vi "nanocal -- nuclear schottky fit V8.vi"() -> ()   [LabVIEW 2021] (continued)
  T36 = typedef "eventvkey.ctl" = enum16{"ASCII", "Enter", "Return", "Shift", "Ctrl", "Alt", "Cmd", "Opt", "Caps", "NumLock", "Clear", "Break", "Up", "Down", "Left", "Right", "Insert", "Delete", "Home", "End", "PageUp", "PageDown", "Escape", "Help", "Pause", "ScrollLock", "F1", "F2", "F3", "F4", "F5", "F6", "F7", "F8", "F9", "F10", "F11", "F12", "F13", "F14", "F15", "F16", "F17", "F18", "F19", "F20", "F21", "F22", "F23", "F24", "Play", "VolumeUp", "VolumeDown", "Mute", "Two Byte Char"}
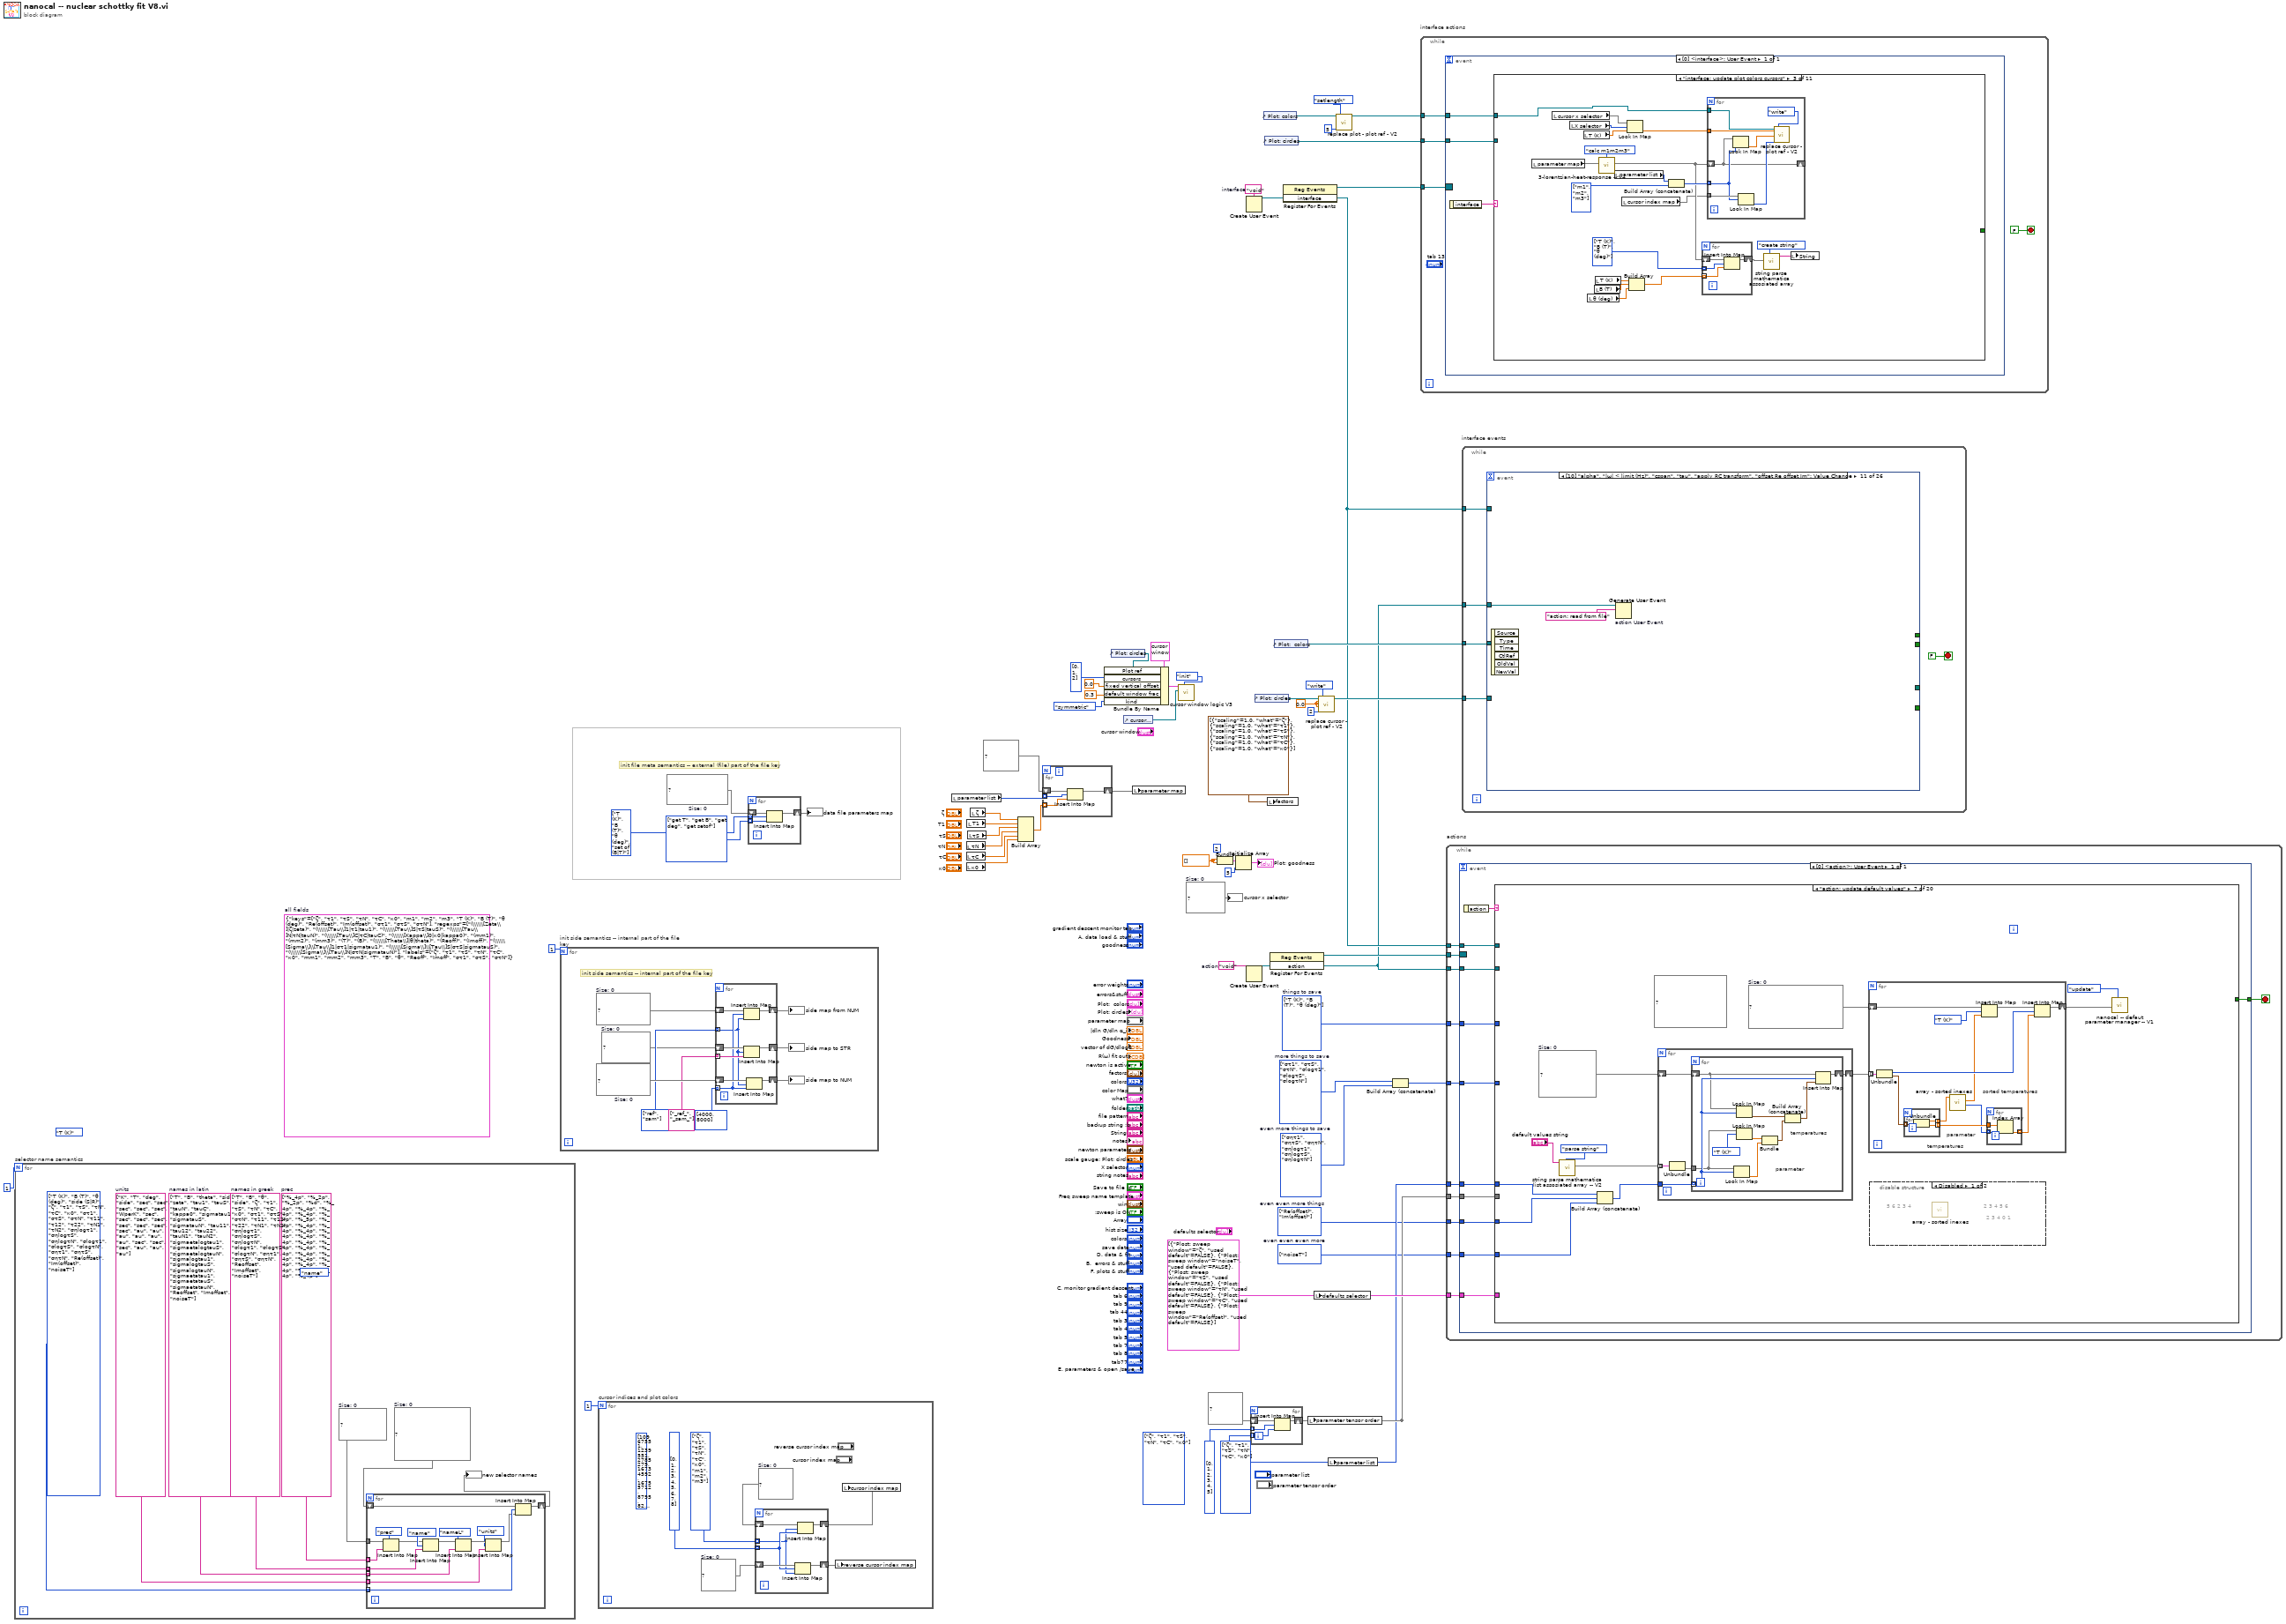
[diagram p0: block diagram]
diagram:
  w2 = T1[] [enum."noiseT"] items=["ζ", "τ1", "τS", "τN", "τC", "κ0", "m1", "m2", "m3", "T (K)", "B (T)", "θ (deg)", "side (S|R)", "set of (B|T)", "Re(offset)", "Im(offset)", "στ1", "στ1-", "στ1+", "στS", "στS-", "στS+", "στN", "στN-", "στN+", "τ11", "τ12", "τ21", "τ22", "τN1", "τN2", "σηlogτ1", "σηlogτS", "σηlogτN", "σlogτ1", "σlogτS", "σlogτN", "σητ1", "σητS", "σητN", "noiseT"]  # even even even more
  (unwired) 3-lorentzian-parameters."T (K)" ("Plost: sweep window")
  w3 = T1[] [enum."Re(offset)", enum."Im(offset)"] items=["ζ", "τ1", "τS", "τN", "τC", "κ0", "m1", "m2", "m3", "T (K)", "B (T)", "θ (deg)", "side (S|R)", "set of (B|T)", "Re(offset)", "Im(offset)", "στ1", "στ1-", "στ1+", "στS", "στS-", "στS+", "στN", "στN-", "στN+", "τ11", "τ12", "τ21", "τ22", "τN1", "τN2", "σηlogτ1", "σηlogτS", "σηlogτN", "σlogτ1", "σlogτS", "σlogτN", "σητ1", "σητS", "σητN", "noiseT"]  # even even more things
  w9 = T1[] [enum."σητ1", enum."σητS", enum."σητN", enum."σηlogτ1", enum."σηlogτS", enum."σηlogτN"] items=["ζ", "τ1", "τS", "τN", "τC", "κ0", "m1", "m2", "m3", "T (K)", "B (T)", "θ (deg)", "side (S|R)", "set of (B|T)", "Re(offset)", "Im(offset)", "στ1", "στ1-", "στ1+", "στS", "στS-", "στS+", "στN", "στN-", "στN+", "τ11", "τ12", "τ21", "τ22", "τN1", "τN2", "σηlogτ1", "σηlogτS", "σηlogτN", "σlogτ1", "σlogτS", "σlogτN", "σητ1", "σητS", "σητN", "noiseT"]  # even more things to save
  w12 = T1[] [enum."ζ", enum."τ1", enum."τS", enum."τN", enum."τC", enum."κ0"] items=["ζ", "τ1", "τS", "τN", "τC", "κ0", "m1", "m2", "m3", "T (K)", "B (T)", "θ (deg)", "side (S|R)", "set of (B|T)", "Re(offset)", "Im(offset)", "στ1", "στ1-", "στ1+", "στS", "στS-", "στS+", "στN", "στN-", "στN+", "τ11", "τ12", "τ21", "τ22", "τN1", "τN2", "σηlogτ1", "σηlogτS", "σηlogτN", "σlogτ1", "σlogτS", "σlogτN", "σητ1", "σητS", "σητN", "noiseT"]
  w16 = T1[] [enum."T (K)", enum."B (T)", enum."θ (deg)"] items=["ζ", "τ1", "τS", "τN", "τC", "κ0", "m1", "m2", "m3", "T (K)", "B (T)", "θ (deg)", "side (S|R)", "set of (B|T)", "Re(offset)", "Im(offset)", "στ1", "στ1-", "στ1+", "στS", "στS-", "στS+", "στN", "στN-", "στN+", "τ11", "τ12", "τ21", "τ22", "τN1", "τN2", "σηlogτ1", "σηlogτS", "σηlogτN", "σlogτ1", "σlogτS", "σlogτN", "σητ1", "σητS", "σητN", "noiseT"]  # things to save
  w11 = T1[] [enum."στ1", enum."στS", enum."στN", enum."σlogτ1", enum."σlogτS", enum."σlogτN"] items=["ζ", "τ1", "τS", "τN", "τC", "κ0", "m1", "m2", "m3", "T (K)", "B (T)", "θ (deg)", "side (S|R)", "set of (B|T)", "Re(offset)", "Im(offset)", "στ1", "στ1-", "στ1+", "στS", "στS-", "στS+", "στN", "στN-", "στN+", "τ11", "τ12", "τ21", "τ22", "τN1", "τN2", "σηlogτ1", "σηlogτS", "σηlogτN", "σlogτ1", "σlogτS", "σlogτN", "σητ1", "σητS", "σητN", "noiseT"]  # more things to save
  (unwired) T16 {"keys"=[enum."ζ", enum."τ1", enum."τS", enum."τN", enum."τC", enum."κ0", enum."m1", enum."m2", enum."m3", enum."T (K)", enum."B (T)", enum."θ (deg)", enum."Re(offset)", enum."Im(offset)", enum."στ1", enum."στS", enum."στN"], "regexps"=["(\\\\\\[Zeta\\]|ζ|zeta)", "(\\\\\\[Tau\\]1|τ1|tau1)", "(\\\\\\[Tau\\]S|τS|tauS)", "(\\\\\\[Tau\\]N|τN|tauN)", "(\\\\\\[Tau\\]C|τC|tauC)", "(\\\\\\[Kappa\\]0|κ0|kappa0)", "(mm1)", "(mm2)", "(mm3)", "(T)", "(B)", "(\\\\\\[Theta\\]|θ|theta)", "(Reoff)", "(Imoff)", "(\\\\\\[Sigma\\]\\[Tau\\]1|στ1|sigmatau1)", "(\\\\\\[Sigma\\]\\[Tau\\]S|στS|sigmatauS)", "(\\\\\\[Sigma\\]\\[Tau\\]N|στN|sigmatauN)"], "labels"=["ζ", "τ1", "τS", "τN", "τC", "κ0", "mm1", "mm2", "mm3", "T", "B", "θ", "Reoff", "Imoff", "στ1", "στS", "στN"]}  # all fields
  (unwired) 2 ("dimension size")
  w33 = T5 [{"Plost: sweep window"=enum."ζ", "used default"=FALSE}, {"Plost: sweep window"=enum."noiseT", "used default"=FALSE}, {"Plost: sweep window"=enum."τS", "used default"=FALSE}, {"Plost: sweep window"=enum."τN", "used default"=FALSE}, {"Plost: sweep window"=enum."τC", "used default"=FALSE}, {"Plost: sweep window"=enum."Re(offset)", "used default"=FALSE}] ("parameter 2")
  w34 = T13[] [enum."get T", enum."get B", enum."get deg", enum."get setof"] items=["rewrite", "parse", "force pattern", "uniquenum", "get T", "get B", "get ind", "get deg", "get name", "get folder", "get extension", "get basename", "get side", "get setof", "getID", "getIDStock"]
  w36 = map{T1, T13} {}  # Size: 0
  w35 = T1[] [enum."T (K)", enum."B (T)", enum."θ (deg)", enum."set of (B|T)"] items=["ζ", "τ1", "τS", "τN", "τC", "κ0", "m1", "m2", "m3", "T (K)", "B (T)", "θ (deg)", "side (S|R)", "set of (B|T)", "Re(offset)", "Im(offset)", "στ1", "στ1-", "στ1+", "στS", "στS-", "στS+", "στN", "στN-", "στN+", "τ11", "τ12", "τ21", "τ22", "τN1", "τN2", "σηlogτ1", "σηlogτS", "σηlogτN", "σlogτ1", "σlogτS", "σlogτN", "σητ1", "σητS", "σητN", "noiseT"]
  w40 = dbl[] []
  (unwired) T1[] [enum."ζ", enum."τ1", enum."τS", enum."τN", enum."τC", enum."κ0"] items=["ζ", "τ1", "τS", "τN", "τC", "κ0", "m1", "m2", "m3", "T (K)", "B (T)", "θ (deg)", "side (S|R)", "set of (B|T)", "Re(offset)", "Im(offset)", "στ1", "στ1-", "στ1+", "στS", "στS-", "στS+", "στN", "στN-", "στN+", "τ11", "τ12", "τ21", "τ22", "τN1", "τN2", "σηlogτ1", "σηlogτS", "σηlogτN", "σlogτ1", "σlogτS", "σlogτN", "σητ1", "σητS", "σητN", "noiseT"]
  w43 = map{T1, dbl} {}  # Size: 0
  w44 = 0.0 ("new X")
  w57 = "void"  # interface
  w58 = "void"  # action
  # "init file meta semantics -- external (file) part of the file key"
  n1 = for "selector name semantics" {
    N: 1 -> [_]
    w60 = string[] ["%_4p", "%_2p", "%_2p", "%d", "%_4p", "%_4p", "%_4p", "%_4p", "%_4p", "%_5p", "%_4p", "%_4p", "%_4p", "%_4p", "%_4p", "%_4p", "%_4p", "%_4p", "%_4p", "%_4p", "%_4p", "%_4p", "%_4p", "%_4p", "%_4p", "%_4p", "%_4p", "%_4p", "%_4p", "%_4p"]  # prec
    w64 = map{T14, string} {}  # Size: 0
    (unwired) nameformattingitem."name" ("name formatting item")
    w62 = string[] ["K", "T", "deg", "side", "sec", "sec", "sec", "sec", "sec", "WperK", "sec", "sec", "sec", "sec", "sec", "sec", "sec", "sec", "au", "au", "au", "au", "au", "au", "sec", "sec", "sec", "au", "au", "au"]  # units
    w65 = string[] ["T", "B", "theta", "side", "zeta", "tau1", "tauS", "tauN", "tauC", "kappa0", "sigmatau1", "sigmatauS", "sigmatauN", "tau11", "tau12", "tau22", "tauN1", "tauN2", "sigmaetalogtau1", "sigmaetalogtauS", "sigmaetalogtauN", "sigmalogtau1", "sigmalogtauS", "sigmalogtauN", "sigmaetatau1", "sigmaetatauS", "sigmaetatauN", "Reoffset", "Imoffset", "noiseT"]  # names in latin
    w63 = string[] ["T", "B", "θ", "side", "ζ", "τ1", "τS", "τN", "τC", "κ0", "στ1", "στS", "στN", "τ11", "τ12", "τ22", "τN1", "τN2", "σηlogτ1", "σηlogτS", "σηlogτN", "σlogτ1", "σlogτS", "σlogτN", "σητ1", "σητS", "σητN", "Reoffset", "Imoffset", "noiseT"]  # names in greek
    w67 = map{T1, map{T14, string}} {}  # Size: 0
    w66 = T1[] [enum."T (K)", enum."B (T)", enum."θ (deg)", enum."side (S|R)", enum."ζ", enum."τ1", enum."τS", enum."τN", enum."τC", enum."κ0", enum."στ1", enum."στS", enum."στN", enum."τ11", enum."τ12", enum."τ22", enum."τN1", enum."τN2", enum."σηlogτ1", enum."σηlogτS", enum."σηlogτN", enum."σlogτ1", enum."σlogτS", enum."σlogτN", enum."σητ1", enum."σητS", enum."σητN", enum."Re(offset)", enum."Im(offset)", enum."noiseT"] items=["ζ", "τ1", "τS", "τN", "τC", "κ0", "m1", "m2", "m3", "T (K)", "B (T)", "θ (deg)", "side (S|R)", "set of (B|T)", "Re(offset)", "Im(offset)", "στ1", "στ1-", "στ1+", "στS", "στS-", "στS+", "στN", "στN-", "στN+", "τ11", "τ12", "τ21", "τ22", "τN1", "τN2", "σηlogτ1", "σηlogτS", "σηlogτN", "σlogτ1", "σlogτS", "σlogτN", "σητ1", "σητS", "σητN", "noiseT"]
    n2 = for {
      shift-right: [w82] -> w61
      shift-left: w67 -> [w83]
      tunnel: w65 -> [w73] mode=indexing
      tunnel: w66 -> [w81] mode=indexing
      tunnel: w64 -> [w71]
      tunnel: w63 -> [w72] mode=indexing
      tunnel: w62 -> [w74] mode=indexing
      tunnel: w60 -> [w70] mode=indexing
      n3 = Insert Into Map(map in=w71, key=nameformattingitem."prec", value=w70) -> (map out=w69:map{T14, string})  [unwired: 2 out]
      n4 = Insert Into Map(map in=w69, key=nameformattingitem."name", value=w72) -> (map out=w80:map{T14, string})  [unwired: 2 out]
      n5 = Insert Into Map(map in=w80, key=nameformattingitem."nameL" ("name formatting item"), value=w73) -> (map out=w79:map{T14, string})  [unwired: 2 out]
      n6 = Insert Into Map(map in=w79, key=nameformattingitem."units" ("name formatting item"), value=w74) -> (map out=w78:map{T14, string})  [unwired: 2 out]
      n7 = Insert Into Map(map in=w83, key=w81, value=w78) -> (map out=w82:map{T1, map{T14, string}})  [unwired: 2 out]
    }
    "new selector names" <- w61
  }
  n8 = for "init side semantics -- internal part of the file key" {
    N: 1 -> [_]
    w85 = map{i32, T9} {}  # Size: 0
    w87 = map{T9, string} {}  # Size: 0
    w88 = T9[] [enum."ref", enum."sam"] items=["sam", "ref"]
    w92 = map{T9, i32} {}  # Size: 0
    # "init side semantics -- internal part of the file key"
    n9 = for {
      shift-right: [w100] -> w89
      shift-left: w92 -> [w101]
      tunnel: string[] ["_ref_", "_sam_"] -> [w97] mode=indexing
      tunnel: i32[] [4000, 8000] -> [w94] mode=indexing
      tunnel: w88 -> [w93] mode=indexing
      shift-right: [w98] -> w86
      shift-left: w87 -> [w99]
      shift-right: [w95] -> w84
      shift-left: w85 -> [w96]
      n10 = Insert Into Map(map in=w96, key=w94, value=w93) -> (map out=w95:map{i32, T9})  [unwired: 2 out]
      n11 = Insert Into Map(map in=w99, key=w93, value=w97) -> (map out=w98:map{T9, string})  [unwired: 2 out]
      n12 = Insert Into Map(map in=w101, key=w93, value=w94) -> (map out=w100:map{T9, i32})  [unwired: 2 out]
    }
    "side map from NUM" <- w84
    "side map to STR" <- w86
    "side map to NUM" <- w89
  }
  n13 = for "cursor indices and plot colors" {
    N: 1 -> [_]
    w103 = map{i32, T1} {}  # Size: 0
    (unwired) u32[] [10967551, 1239551, 2785279, 16734592, 16755712, 8795, 8285330, 9272482, 9204890]
    w107 = map{T1, i32} {}  # Size: 0
    w104 = T1[] [enum."ζ", enum."τ1", enum."τS", enum."τN", enum."τC", enum."κ0", enum."m1", enum."m2", enum."m3"] items=["ζ", "τ1", "τS", "τN", "τC", "κ0", "m1", "m2", "m3", "T (K)", "B (T)", "θ (deg)", "side (S|R)", "set of (B|T)", "Re(offset)", "Im(offset)", "στ1", "στ1-", "στ1+", "στS", "στS-", "στS+", "στN", "στN-", "στN+", "τ11", "τ12", "τ21", "τ22", "τN1", "τN2", "σηlogτ1", "σηlogτS", "σηlogτN", "σlogτ1", "σlogτS", "σlogτN", "σητ1", "σητS", "σητN", "noiseT"]
    n14 = for {
      shift-right: [w112] -> w105
      shift-left: w107 -> [w113]
      tunnel: w104 -> [w108] mode=indexing
      tunnel: i32[] [0, 1, 2, 3, 4, 5, 6, 7, 8] -> [w109] mode=indexing
      shift-right: [w110] -> w102
      shift-left: w103 -> [w111]
      n15 = Insert Into Map(map in=w111, key=w109, value=w108) -> (map out=w110:map{i32, T1})  [unwired: 2 out]
      n16 = Insert Into Map(map in=w113, key=w108, value=w109) -> (map out=w112:map{T1, i32})  [unwired: 2 out]
    }
    n17 = local write "reverse cursor index map"(w102) -> ()
    n18 = local write "cursor index map"(w105) -> ()
  }
  n19 = for {
    shift-right: [w116] -> w37
    shift-left: w36 -> [w117]
    tunnel: w35 -> [w115] mode=indexing
    tunnel: w34 -> [w114] mode=indexing
    n20 = Insert Into Map(map in=w117, key=w115, value=w114) -> (map out=w116:map{T1, T13})  [unwired: 2 out]
  }
  "data file parameters map" <- w37
  n21 = local read "parameter list"() -> (w1:T1[])
  n22 = local read "τN"() -> (w25:dbl)
  n23 = local read "τC"() -> (w26:dbl)
  n24 = local read "κ0"() -> (w27:dbl)
  n25 = local read "T1"() -> (w23:dbl)
  n26 = local read "τS"() -> (w24:dbl)
  n27 = local read "ζ"() -> (w22:dbl)
  n28 = Build Array(w22, w23, w24, w25, w26, w27) -> (w28:dbl[])
  n29 = for {
    shift-right: [w120] -> w29
    shift-left: map{T1, dbl} {} ("Map IN") -> [w121]
    tunnel: w1 -> [w119] mode=indexing
    tunnel: w28 -> [w118] mode=indexing
    n30 = Insert Into Map(map in=w121, key=w119, value=w118) -> (map out=w120:map{T1, dbl})  [unwired: 2 out]
  }
  n31 = control-ref of="Plot: circles"() -> (w49:refnum<vi>)
  n32 = Bundle By Name(cluster=T12 {"left"=0.0, "right "=0.0, "center"=0.0, "window"=0.0, "cursors"=[], "relative"=0, "absolute"=0, "fixed vertical offset"=0.0, "vertical offset"=0.0, "skew"=0.0, "default window frac"=0.0, "kind"=enum."symmetric", "skew.left"=0.0, "skew.right"=0.0, "Plot ref"=refnum, "wing order"=enum."forw"} ("cursor bracket: All, data window"), "Plot ref"=w49, "cursors"=i32[] [0, 1, 2], "fixed vertical offset"=0.0, "default window frac"=0.3 ("fixed vertical offset"), "kind"=enum16{"symmetric", "skewed", "fancy"}."symmetric") -> (w52:T12)
  n33 = control-ref of="cursor window"() -> (w48:refnum<vi>)
  n34 = local write "parameter map"(w29) -> ()
  n35 = call "cursor window logic V3.vi"("cursor window action"=cursor_window_action."init", "cursor window in"=w48, "cursor window init"=w52) -> ()  [unwired: 7 in, 2 out]
  n36 = Bundle(w40, w40) -> (w17:cluster{dbl[], dbl[]})  [unwired: 1 in]
  n37 = Initialize Array(w17, 5 ("dimension size")) -> (→"Plot: goodness":cluster{dbl[], dbl[]}[])
  n38 = Create User Event(user event datatype=w57) -> (user event=w19:refnum<user-event>)  [unwired: 1 in, 1 out]
  n39 = Create User Event(user event datatype=w58) -> (user event=w18:refnum<user-event>)  [unwired: 1 in, 1 out]
  n40 = for {
    tunnel: w12 -> [w122] mode=indexing
    shift-right: [w124] -> w13
    shift-left: map{i32, T1} {} ("parameters IN") -> [w125]
    tunnel: i32[] [0, 1, 2, 3, 4, 5] -> [w123] mode=indexing
    n41 = Insert Into Map(map in=w125, key=w123, value=w122) -> (map out=w124:map{i32, T1})  [unwired: 2 out]
  }
  n42 = control-ref of="Plot: circles"() -> (w45:refnum<vi>)
  n43 = control-ref of="Plot: colors"() -> (w5:refnum<vi>)
  n44 = control-ref of="Plot: circles"() -> (w6:refnum<vi>)
  n45 = local write "factors"(cluster{"scaling":dbl, "what":T1}[] [{"scaling"=1.0, "what"=enum."ζ"}, {"scaling"=1.0, "what"=enum."τ1"}, {"scaling"=1.0, "what"=enum."τS"}, {"scaling"=1.0, "what"=enum."τN"}, {"scaling"=1.0, "what"=enum."τC"}, {"scaling"=1.0, "what"=enum."κ0"}]) -> ()
  n46 = register-events(w18) -> (reference out=w59:refnum<event-registration>)  [unwired: 2 in, 1 out]
  n47 = control-ref of="Plot:  colors"() -> (w42:refnum<vi>)
  n48 = register-events(w19) -> (reference out=w20:refnum<event-registration>)  [unwired: 2 in, 1 out]
  n49 = local write "parameter tensor order"(w13) -> ()
  n50 = local write "defaults selector"(w33) -> ()
  n51 = call "replace cursor - plot ref - V2.vi"("Plot ref in"=w45, "new X"=w44, "new  Y"=w44, "cursor index"=2, "cursor action"=cursor_action."write") -> ()  [unwired: 11 in, 4 out]
  n52 = local write "parameter list"(w12) -> ()
  n53 = call "replace plot - plot ref - V2.vi"("Plot ref in"=w5, "plot index"=5, "cursor action"=cursor_action."setlength") -> ("Plot ref out"=w4:refnum<vi>)  [unwired: 12 in, 4 out]
  n54 = Build Array (concatenate)(w11, w9) -> (w10:T1[])
  n55 = while "interface actions" {
    tunnel: w20 -> [w129]
    tunnel: w4 -> [w128]
    tunnel: w6 -> [w127]
    stop <- FALSE stop-if-true
    n56 = event shown="[0] <interface>: User Event" {
      selector: w129 -> [_]
      dyn-events: _ -> [_]
      timeout: _ -> [_]
      tunnel: w128 -> [w131]
      tunnel: w127 -> [w130]
      event User Event {
        n57 = event-data() -> ("interface"=w132:string)  [unwired: 1 in]
        n58 = case shown="\"interface: update plot colors cursors\"" w132 {
          tunnel: [_ _ _ _ _ _ _ _ _ _ TRUE] -> _
          tunnel: w131 -> [_ _ w153 w185 _ _ w236 w307 _ _ _]
          tunnel: w130 -> [_ _ _ _ w203 _ _ _ _ _ _]
          frame "void", Default {
          }
          frame "interface: reset colors" {
            w139 = map{T1, u32} {}  # Size: 0
            n59 = local read "parameter list"() -> (w142:T1[])
            n60 = local read "colors"() -> (w140:u32[])
            n61 = for {
              shift-right: [w151] -> w141
              shift-left: w139 -> [w152]
              tunnel: w142 -> [w150] mode=indexing
              tunnel: w140 -> [w149] mode=indexing
              n62 = Insert Into Map(map in=w152, key=w150, value=w149) -> (map out=w151:map{T1, u32})  [unwired: 2 out]
            }
            n63 = local write "color Map"(w141) -> ()
            n64 = Look In Map(map=w141, key=3-lorentzian-parameters."ζ" ("Plost: sweep window")) -> (value=w143:u32)  [unwired: 1 in, 1 out]
            n65 = Look In Map(map=w141, key=3-lorentzian-parameters."τ1" ("Plost: sweep window")) -> (value=w144:u32)  [unwired: 1 in, 1 out]
            n66 = Look In Map(map=w141, key=3-lorentzian-parameters."τS" ("Plost: sweep window")) -> (value=w145:u32)  [unwired: 1 in, 1 out]
            n67 = Look In Map(map=w141, key=3-lorentzian-parameters."τN" ("Plost: sweep window")) -> (value=w146:u32)  [unwired: 1 in, 1 out]
            n68 = Look In Map(map=w141, key=3-lorentzian-parameters."τC" ("Plost: sweep window")) -> (value=w147:u32)  [unwired: 1 in, 1 out]
            n69 = Look In Map(map=w141, key=3-lorentzian-parameters."κ0" ("Plost: sweep window")) -> (value=w148:u32)  [unwired: 1 in, 1 out]
            n70 = property on="ζ" class="Slide (strict)"("Fill Color"=w143) -> ()  [unwired: 2 in, 2 out]
            n71 = property on="T1" class="Slide (strict)"("Fill Color"=w144) -> ()  [unwired: 2 in, 2 out]
            n72 = property on="τS" class="Slide (strict)"("Fill Color"=w145) -> ()  [unwired: 2 in, 2 out]
            n73 = property on="τN" class="Slide (strict)"("Fill Color"=w146) -> ()  [unwired: 2 in, 2 out]
            n74 = property on="τC" class="Slide (strict)"("Fill Color"=w147) -> ()  [unwired: 2 in, 2 out]
            n75 = property on="κ0" class="Slide (strict)"("Fill Color"=w148) -> ()  [unwired: 2 in, 2 out]
          }
          frame "interface: update plot colors cursors" {
            w158 = T1[] [enum."m1", enum."m2", enum."m3"] items=["ζ", "τ1", "τS", "τN", "τC", "κ0", "m1", "m2", "m3", "T (K)", "B (T)", "θ (deg)", "side (S|R)", "set of (B|T)", "Re(offset)", "Im(offset)", "στ1", "στ1-", "στ1+", "στS", "στS-", "στS+", "στN", "στN-", "στN+", "τ11", "τ12", "τ21", "τ22", "τN1", "τN2", "σηlogτ1", "σηlogτS", "σηlogτN", "σlogτ1", "σlogτS", "σlogτN", "σητ1", "σητS", "σητN", "noiseT"]
            w156 = T1[] [enum."T (K)", enum."B (T)", enum."θ (deg)"] items=["ζ", "τ1", "τS", "τN", "τC", "κ0", "m1", "m2", "m3", "T (K)", "B (T)", "θ (deg)", "side (S|R)", "set of (B|T)", "Re(offset)", "Im(offset)", "στ1", "στ1-", "στ1+", "στS", "στS-", "στS+", "στN", "στN-", "στN+", "τ11", "τ12", "τ21", "τ22", "τN1", "τN2", "σηlogτ1", "σηlogτS", "σηlogτN", "σlogτ1", "σlogτS", "σlogτN", "σητ1", "σητS", "σητN", "noiseT"]
            n76 = local read "parameter map"() -> (w171:map{T1, dbl})
            n77 = local read "cursor x selector"() -> (w159:map{T1, dbl})
            n78 = local read "X selector"() -> (w160:T1)
            n79 = local read "T (K)"() -> (w161:dbl)
            n80 = local read "θ (deg)"() -> (w166:dbl)
            n81 = local read "B (T)"() -> (w165:dbl)
            n82 = local read "T (K)"() -> (w164:dbl)
            n83 = call "3-lorentzian-heat-response -- V4.vi"("action"=3-lorentzian-heat-response_action."calc m1m2m3", "Map IN"=w171) -> ("Map OUT"=w167:map{T1, dbl})  [unwired: 7 in, 2 out]
            n84 = local read "parameter list"() -> (w172:T1[])
            n85 = local read "cursor index map"() -> (w163:map{T1, i32})
            n86 = Look In Map(map=w159, key=w160, default value=w161) -> (value=w162:dbl)  [unwired: 1 out]
            n87 = Build Array(w164, w165, w166) -> (w154:dbl[])
            n88 = Build Array (concatenate)(w172, w158) -> (w170:T1[])
            n89 = for {
              shift-right: [w175] -> w168
              shift-left: w167 -> [w176]
              tunnel: w156 -> [w174] mode=indexing
              tunnel: w154 -> [w173] mode=indexing
              n90 = Insert Into Map(map in=w176, key=w174, value=w173) -> (map out=w175:map{T1, dbl})  [unwired: 2 out]
            }
            n91 = for {
              tunnel: w162 -> [w184]
              tunnel: w153 -> [w183]
              tunnel: w170 -> [w179] mode=indexing
              tunnel: w163 -> [w181]
              shift-right: [w178] -> _
              shift-left: w167 -> [w178]
              n92 = Look In Map(map=w178, key=w179) -> (value=w177:dbl)  [unwired: 1 in, 1 out]
              n93 = Look In Map(map=w181, key=w179) -> (value=w180:i32)  [unwired: 1 in, 1 out]
              n94 = call "replace cursor - plot ref - V2.vi"("Plot ref in"=w183, "new X"=w184, "new  Y"=w177, "cursor index"=w180, "cursor action"=cursor_action."write") -> ()  [unwired: 11 in, 4 out]
            }
            n95 = call "string parse mathematica assosiated array.vi"("action"=mathematica_string_map_action."create string" ("derivative"), "map IN"=w168) -> ("String OUT"=w169:string)  [unwired: 8 in, 1 out]
            n96 = local write "String"(w169) -> ()
          }
          frame "interface: plot colors update m1m2m3 cursors" {
            w186 = T1[] [enum."m1", enum."m2", enum."m3"] items=["ζ", "τ1", "τS", "τN", "τC", "κ0", "m1", "m2", "m3", "T (K)", "B (T)", "θ (deg)", "side (S|R)", "set of (B|T)", "Re(offset)", "Im(offset)", "στ1", "στ1-", "στ1+", "στS", "στS-", "στS+", "στN", "στN-", "στN+", "τ11", "τ12", "τ21", "τ22", "τN1", "τN2", "σηlogτ1", "σηlogτS", "σηlogτN", "σlogτ1", "σlogτS", "σlogτN", "σητ1", "σητS", "σητN", "noiseT"]
            n97 = local read "parameter map"() -> (w194:map{T1, dbl})
            n98 = call "3-lorentzian-heat-response -- V4.vi"("action"=3-lorentzian-heat-response_action."calc m1m2m3", "Map IN"=w194) -> ("Map OUT"=w193:map{T1, dbl})  [unwired: 7 in, 2 out]
            n99 = local read "cursor x selector"() -> (w188:map{T1, dbl})
            n100 = local read "X selector"() -> (w189:T1)
            n101 = local read "cursor index map"() -> (w192:map{T1, i32})
            n102 = local read "T (K)"() -> (w190:dbl)
            n103 = Look In Map(map=w188, key=w189, default value=w190) -> (value=w191:dbl)  [unwired: 1 out]
            n104 = for {
              tunnel: w191 -> [w202]
              tunnel: w186 -> [w198] mode=indexing
              tunnel: w192 -> [w200]
              shift-right: [w197] -> _
              shift-left: w193 -> [w197]
              tunnel: w185 -> [w195]
              n105 = Look In Map(map=w197, key=w198) -> (value=w196:dbl)  [unwired: 1 in, 1 out]
              n106 = Look In Map(map=w200, key=w198) -> (value=w199:i32)  [unwired: 1 in, 1 out]
              n107 = call "replace cursor - plot ref - V2.vi"("Plot ref in"=w195, "new X"=w202, "new  Y"=w196, "cursor index"=w199, "cursor action"=cursor_action."write") -> ()  [unwired: 11 in, 4 out]
            }
          }
          frame "interface: update circle fit plot" {
            n108 = for {
              N: 1 -> [_]
              tunnel: w203 -> [w206]
              n109 = local read "update  ind"() -> (w208:i32)
              n110 = local read "vector of dG/dlogα"() -> (w210:dbl[])
              n111 = Increment(x=w208) -> (x+1=w207:i32)
              n112 = local read "R(ω) fit out"() -> (w216:cdb[])
              n113 = Square(x=w210) -> (x^2=w205:dbl[])
              n114 = local write "update  ind"(w207) -> ()
              n115 = Complex To Re/Im(x + iy=w216) -> (x=w214:dbl[], y=w215:dbl[])
              n116 = Add Array Elements(numeric array=w205) -> (sum=w211:dbl)
              n117 = call "replace plot - plot ref - V2.vi"("Plot ref in"=w206, "Array X IN"=w214, "Array Y IN"=w215, "plot index"=enum16{"data R(ω)", "fit R(ω)"}."fit R(ω)" ("Plost: sweep window"), "cursor action"=cursor_action."write") -> ()  [unwired: 10 in, 5 out]
              n118 = Square Root(x=w211) -> (sqrt(x)=w209:dbl)
              n119 = local write "|dln G/dln α_i |"(w209) -> ()
            }
          }
          frame "interface: update curvature plot" {
            n120 = local read "newton parameters"() -> (w219:T2)
            n121 = local read "error weights"() -> (w218:T4)
            n122 = Bundle By Name(cluster=w219, "weighting"=w218) -> (w217:T2)
            n123 = case shown="True" "update errors as you fit" {
              tunnel: w217 -> [_ w225]
              frame False {
              }
              frame True {
                n124 = local read "parameter tensor order"() -> (w221:map{i32, T1})
                n125 = local read "errors&stuff"() -> (w226:T10)
                n126 = local read "parameter map"() -> (w228:map{T1, dbl})
                n127 = local read "parameter list"() -> (w222:T1[])
                n128 = call "nanocal -- publish -- freq scan V2.vi"("publisher action"=publisher_action."get") -> ("data"=w223:T21)  [unwired: 7 in, 3 out]
                n129 = call "nanocal -- generate 3D curvature ellipsoid --  V5.vi"("parameter keys IN"=w222, "parameter tensor order IN"=w221, "parameters IN"=w228, "data IN"=w223, "errors IN"=w226, "newton parameters"=w225) -> ("errors pair OUT"=w224:T10)  [unwired: 9 in]
                n130 = local write "errors&stuff"(w224) -> ()
              }
            }
          }
          frame "interface: replot colors plot" {
            n131 = local read "X selector"() -> (w237:T1)
            n132 = local read "color data"() -> (w231:cluster{"Array":dbl[], "Array":dbl[]}[])
            n133 = local read "cursor index map"() -> (w238:map{T1, i32})
            n134 = case shown="\"B (T)\"" w237 {
              tunnel: ["B (T)" "T (K)"] -> w242
              frame "B (T)" {
              }
              frame "T (K)", Default {
              }
            }
            n135 = local read "parameter list"() -> (w243:T1[])
            n136 = local read "color Map"() -> (w239:map{T1, u32})
            n137 = call "replace plot - plot ref - V2.vi"("Plot ref in"=w236, "text"=w242, "cursor action"=cursor_action."set Xlabel") -> ("Plot ref out"=w240:refnum<vi>)  [unwired: 12 in, 4 out]
            n138 = for {
              tunnel: w243 -> [w288] mode=indexing
              tunnel: w231 -> [w286] mode=indexing
              tunnel: w239 -> [w283]
              tunnel: w238 -> [w282]
              shift-right: [w281] -> w234
              shift-left: w240 -> [w287]
              shift-right: [w279] -> w229
              shift-left: i64 0 -> [w280]
              n139 = Unbundle(w286) -> ("Array"=w284:dbl[], "Array"=w285:dbl[])
              n140 = case shown="\"ζ\"..\"τC\", Default" w288 {
                selector: w288 -> [_ w302]
                tunnel: w284 -> [_ w304]
                tunnel: w285 -> [_ w303]
                tunnel: w283 -> [_ w301]
                tunnel: w282 -> [_ w300]
                tunnel: w287 -> [w290 w295]
                tunnel: [w290 w293] -> w281
                tunnel: w280 -> [w289 w292]
                tunnel: [w289 w291] -> w279
                frame "κ0" {
                }
                frame "ζ".."τC", Default {
                  n141 = Look In Map(map=w300, key=w302) -> (value=w294:i32)  [unwired: 1 in, 1 out]
                  n142 = call "replace plot - plot ref - V2.vi"("Plot ref in"=w295, "Array X IN"=w304, "Array Y IN"=w303, "plot index"=w294, "cursor action"=cursor_action."write") -> ("Plot ref out"=w299:refnum<vi>)  [unwired: 10 in, 4 out]
                  n143 = Look In Map(map=w301, key=w302) -> (value=w296:u32)  [unwired: 1 in, 1 out]
                  n144 = call "replace cursor - plot ref - V2.vi"("Plot ref in"=w299, "cursor index"=w294, "cursor action"=cursor_action."set cursor color", "Color Box"=w296) -> ("Plot ref out"=w298:refnum<vi>)  [unwired: 12 in, 3 out]
                  n145 = Increment(x=w292) -> (x+1=w291:i64)
                  n146 = call "replace plot - plot ref - V2.vi"("Plot ref in"=w298, "plot index"=w294, "cursor action"=cursor_action."set plot color", "Color Box"=w296) -> ("Plot ref out"=w293:refnum<vi>)  [unwired: 11 in, 4 out]
                }
              }
            }
            n147 = Empty Collection?(1:"plotme waves") -> (0:w235:bool)
            n148 = case shown="False" w235 {
              tunnel: w234 -> [w244 w270]
              tunnel: "plotme waves" -> [w249 _]
              tunnel: "T" ("key") -> [w247 _]
              tunnel: w229 -> [w245 w267]
              frame False {
                (unwired) 0 ("Numeric OUT")
                n149 = Remove From Map(10:w247, 11:w249) -> (1:w246:dbl[], 3:w248:map{string, dbl[]})  [unwired: 1 out]
                n150 = for {
                  shift-right: [w254] -> _
                  shift-left: w245 -> [w253]
                  tunnel: w248 -> [w264] mode=indexing
                  shift-right: [w263] -> _
                  shift-left: w246 -> [w263]
                  shift-right: [w259] -> _
                  shift-left: w244 -> [w251]
                  w257 = u32 7697781 ("Color Box")
                  n151 = Unbundle(w264) -> ("header OUT"=w261:string, w262:dbl[])
                  n152 = call "replace plot - plot ref - V2.vi"("Plot ref in"=w251, "plot index"=w253, "cursor action"=cursor_action."extend +1 if short") -> ("Plot ref out"=w250:refnum<vi>)  [unwired: 12 in, 4 out]
                  n153 = call "replace plot - plot ref - V2.vi"("Plot ref in"=w250, "plot index"=w253, "cursor action"=cursor_action."unhide plot") -> ("Plot ref out"=w256:refnum<vi>)  [unwired: 12 in, 4 out]
                  n154 = call "replace plot - plot ref - V2.vi"("Plot ref in"=w256, "Array X IN"=w263, "Array Y IN"=w262, "text"=w261, "plot index"=w253, "cursor action"=cursor_action."write", "Color Box"=w257) -> ("Plot ref out"=w260:refnum<vi>)  [unwired: 8 in, 4 out]
                  n155 = Increment(x=w253) -> (x+1=w254:i64)
                  n156 = call "replace plot - plot ref - V2.vi"("Plot ref in"=w260, "plot index"=w253, "cursor action"=cursor_action."set plot color", "Color Box"=w257) -> ("Plot ref out"=w259:refnum<vi>)  [unwired: 11 in, 4 out]
                }
              }
              frame True {
                n157 = call "replace plot - plot ref - V2.vi"("Plot ref in"=w270, "cursor action"=cursor_action."checklngth") -> ("Plot ref out"=w269:refnum<vi>, "Numeric OUT"=w268:i32)  [unwired: 13 in, 3 out]
                n158 = Subtract(x=w268, y=w267) -> (x-y=w266:i64)
                n159 = for {
                  N: w266 -> [_]
                  shift-right: [w274] -> _
                  shift-left: w267 -> [w272]
                  shift-right: [w273] -> _
                  shift-left: w269 -> [w276]
                  n160 = Increment(x=w272) -> (x+1=w274:i64)
                  n161 = call "replace plot - plot ref - V2.vi"("Plot ref in"=w276, "plot index"=w272, "cursor action"=cursor_action."hide plot") -> ("Plot ref out"=w273:refnum<vi>)  [unwired: 12 in, 4 out]
                }
              }
            }
          }
          frame "interface: update color cursors" {
            w309 = T1[] [enum."ζ", enum."τ1", enum."τS", enum."τN", enum."τC", enum."κ0", enum."m1", enum."m2", enum."m3"] items=["ζ", "τ1", "τS", "τN", "τC", "κ0", "m1", "m2", "m3", "T (K)", "B (T)", "θ (deg)", "side (S|R)", "set of (B|T)", "Re(offset)", "Im(offset)", "στ1", "στ1-", "στ1+", "στS", "στS-", "στS+", "στN", "στN-", "στN+", "τ11", "τ12", "τ21", "τ22", "τN1", "τN2", "σηlogτ1", "σηlogτS", "σηlogτN", "σlogτ1", "σlogτS", "σlogτN", "σητ1", "σητS", "σητN", "noiseT"]
            n162 = local read "cursor x selector"() -> (w311:map{T1, dbl})
            n163 = local read "parameter map"() -> (w308:map{T1, dbl})
            n164 = local read "X selector"() -> (w312:T1)
            n165 = local read "T (K)"() -> (w313:dbl)
            n166 = Look In Map(map=w311, key=w312, default value=w313) -> (value=w314:dbl)  [unwired: 1 out]
            n167 = local read "cursor index map"() -> (w315:map{T1, i32})
            n168 = call "3-lorentzian-heat-response -- V4.vi"("action"=3-lorentzian-heat-response_action."calc m1m2m3", "Map IN"=w308) -> ("Map OUT"=w316:map{T1, dbl})  [unwired: 7 in, 2 out]
            n169 = for {
              tunnel: w314 -> [w324]
              tunnel: w307 -> [w323]
              tunnel: w309 -> [w319] mode=indexing
              tunnel: w315 -> [w321]
              shift-right: [w318] -> _
              shift-left: w316 -> [w318]
              n170 = Look In Map(map=w318, key=w319) -> (value=w317:dbl)  [unwired: 1 in, 1 out]
              n171 = Look In Map(map=w321, key=w319) -> (value=w320:i32)  [unwired: 1 in, 1 out]
              n172 = call "replace cursor - plot ref - V2.vi"("Plot ref in"=w323, "new X"=w324, "new  Y"=w317, "cursor index"=w320, "cursor action"=cursor_action."write") -> ()  [unwired: 11 in, 4 out]
            }
          }
          frame "interface: update fit string" {
            w327 = T1[] [enum."T (K)", enum."B (T)", enum."θ (deg)"] items=["ζ", "τ1", "τS", "τN", "τC", "κ0", "m1", "m2", "m3", "T (K)", "B (T)", "θ (deg)", "side (S|R)", "set of (B|T)", "Re(offset)", "Im(offset)", "στ1", "στ1-", "στ1+", "στS", "στS-", "στS+", "στN", "στN-", "στN+", "τ11", "τ12", "τ21", "τ22", "τN1", "τN2", "σηlogτ1", "σηlogτS", "σηlogτN", "σlogτ1", "σlogτS", "σlogτN", "σητ1", "σητS", "σητN", "noiseT"]
            n173 = local read "parameter map"() -> (w325:map{T1, dbl})
            n174 = local read "θ (deg)"() -> (w331:dbl)
            n175 = local read "B (T)"() -> (w330:dbl)
            n176 = local read "T (K)"() -> (w329:dbl)
            n177 = call "3-lorentzian-heat-response -- V4.vi"("action"=3-lorentzian-heat-response_action."calc m1m2m3", "Map IN"=w325) -> ("Map OUT"=w332:map{T1, dbl})  [unwired: 7 in, 2 out]
            n178 = Build Array(w329, w330, w331) -> (w333:dbl[])
            n179 = for {
              shift-right: [w338] -> w334
              shift-left: w332 -> [w339]
              tunnel: w327 -> [w337] mode=indexing
              tunnel: w333 -> [w336] mode=indexing
              n180 = Insert Into Map(map in=w339, key=w337, value=w336) -> (map out=w338:map{T1, dbl})  [unwired: 2 out]
            }
            n181 = call "string parse mathematica assosiated array.vi"("action"=mathematica_string_map_action."create string" ("derivative"), "map IN"=w334) -> ("String OUT"=w335:string)  [unwired: 8 in, 1 out]
            n182 = local write "String"(w335) -> ()
          }
          frame "interface: update list from parameter map" {
            w341 = T1[] [enum."ζ", enum."τ1", enum."τS", enum."τN", enum."τC", enum."κ0"] items=["ζ", "τ1", "τS", "τN", "τC", "κ0", "m1", "m2", "m3", "T (K)", "B (T)", "θ (deg)", "side (S|R)", "set of (B|T)", "Re(offset)", "Im(offset)", "στ1", "στ1-", "στ1+", "στS", "στS-", "στS+", "στN", "στN-", "στN+", "τ11", "τ12", "τ21", "τ22", "τN1", "τN2", "σηlogτ1", "σηlogτS", "σηlogτN", "σlogτ1", "σlogτS", "σlogτN", "σητ1", "σητS", "σητN", "noiseT"]
            n183 = local read "parameter map"() -> (w344:map{T1, dbl})
            n184 = Array Size(array=w341) -> (size(s)=w340:i32)
            n185 = Initialize Array(0.0 ("new X"), w340) -> (w343:dbl[])
            n186 = for {
              tunnel: w341 -> [w362] mode=indexing
              tunnel: w344 -> [w363]
              shift-right: [w360] -> w346
              shift-left: w343 -> [w361]
              i -> [w359]
              n187 = Look In Map(map=w363, key=w362) -> (value=w358:dbl)  [unwired: 1 in, 1 out]
              n188 = Replace Array Subset(array=w361, new element=w358, index=w359) -> (w360:dbl[])
            }
            n189 = Index Array(array=w346, index #1=0 ("index"), index #2=1 ("index"), index #3=2 ("index"), index #4=3 ("index"), index #5=4 ("index"), index #6=5 ("index")) -> (element #1=w345:dbl, element #2=w353:dbl, element #3=w354:dbl, element #4=w355:dbl, element #5=w356:dbl, element #6=w357:dbl)
            n190 = local write "ζ"(w345) -> ()
            n191 = local write "τS"(w354) -> ()
            n192 = local write "τN"(w355) -> ()
            n193 = local write "τC"(w356) -> ()
            n194 = local write "κ0"(w357) -> ()
            n195 = local write "T1"(w353) -> ()
          }
          frame "interface: exit" {
          }
        }
      }
    }
  }
  n196 = while "actions" {
    tunnel: w59 -> [w375]
    tunnel: w18 -> [w374]
    tunnel: w19 -> [w372]
    tunnel: w12 -> [w371]
    tunnel: w33 -> [w370]
    tunnel: w10 -> [w369]
    tunnel: w16 -> [w368]
    tunnel: w13 -> [w367]
    tunnel: w3 -> [w366]
    tunnel: w2 -> [w365]
    stop <- w373 stop-if-true
    n197 = event shown="[0] <action>: User Event" {
      selector: w375 -> [_]
      dyn-events: _ -> [_]
      timeout: _ -> [_]
      tunnel: w374 -> [w385]
      tunnel: [w384] -> w373
      tunnel: w372 -> [w383]
      tunnel: w371 -> [w382]
      tunnel: w370 -> [w381]
      tunnel: w369 -> [w380]
      tunnel: w368 -> [w379]
      tunnel: w367 -> [w378]
      tunnel: w366 -> [w377]
      tunnel: w365 -> [w376]
      event User Event {
        n198 = event-data() -> ("action"=w386:string)  [unwired: 1 in]
        n199 = case shown="\"action: update default values\"" w386 {
          tunnel: w385 -> [w394 _ _ _ w609 w634 _ _ w830 _ w957 _ _ w1065 w1126 w1241 _ w1310 _ _]
          tunnel: [_ _ _ _ _ _ _ _ _ _ _ _ _ _ _ _ TRUE _ _ _] -> w384
          tunnel: w383 -> [w397 w402 _ w531 w603 _ _ _ _ _ _ _ w975 _ w1118 _ _ _ _ _]
          tunnel: w382 -> [_ w409 w419 w530 _ _ w764 _ _ _ _ _ w973 _ w1122 w1216 _ _ _ _]
          tunnel: w381 -> [_ _ _ _ _ _ _ _ _ _ _ _ _ _ _ _ _ _ _ _]
          tunnel: w380 -> [_ _ _ _ _ _ _ _ _ _ _ _ w971 _ _ w1222 _ _ _ _]
          tunnel: w379 -> [_ _ _ _ _ _ _ _ _ _ _ _ _ _ _ w1220 _ _ _ _]
          tunnel: w378 -> [_ w400 w416 w526 _ _ _ _ _ _ _ _ _ _ _ w1215 _ _ _ _]
          tunnel: w377 -> [_ _ _ _ _ _ w763 _ _ _ _ _ w970 _ w1117 w1208 _ _ _ _]
          tunnel: w376 -> [_ _ _ _ _ _ w761 _ _ _ _ _ w969 _ w1114 w1207 _ _ _ _]
          frame "action: new sweep" {
            n200 = Generate User Event(user event=w397, event data cluster="interface: update plot colors cursors" ("event data")) -> (user event out=w398:refnum<user-event>)  [unwired: 2 in, 1 out]
            n201 = Generate User Event(user event=w398, event data cluster="interface: reset colors" ("event data")) -> ()  [unwired: 2 in, 2 out]
            n202 = Generate User Event(user event=w394, event data cluster="action: replot circles" ("event data")) -> ()  [unwired: 2 in, 2 out]
            n203 = call "nanocal -- publish -- freq scan V2.vi"("publisher action"=publisher_action."get") -> ("z out (V)"=w393:cdb[])  [unwired: 7 in, 3 out]
            n204 = control-ref of="Plot: circles"() -> (w388:refnum<vi>)
            n205 = Complex To Re/Im(x + iy=w393) -> (x=w391:dbl[], y=w392:dbl[])
